vi "IO Test.vi"() -> ()   [LabVIEW 2016]
uses:
  <vilib>/rvi/Emulation/niFpgaGetClockAttributes.vi
  <vilib>/rvi/Emulation/niFpgaSctlEmulationGetInTimedLoop.vi
  <vilib>/rvi/Emulation/niFpgaEmulationReportErrorSimple.vi
  <vilib>/rvi/Emulation/niFpgaEmulationIsFPGAContextNoSignature.vi
  <vilib>/rvi/DataTransferAndStorage/Container/Common/niFpgaContainerGetUniqueNameForEmu.vi
  <vilib>/rvi/Memory/Memory_Emulation/niFpgaMemoryEmulationCacheClearOnFirstRun.vi
  <vilib>/rvi/Memory/Memory_Emulation/nirvimemoryEmulationManagerCache_MakeExclusive.vi
  <vilib>/rvi/Memory/Memory_Emulation/niFpgaMemoryEmulationValidateCache.vi
  <vilib>/rvi/Memory/Memory_Emulation/nirvimemoryEmulationManagerCache_InsertValue.vi
  <vilib>/Utility/error.llb/Clear Errors.vi
  <vilib>/rvi/Memory/Memory_Emulation/nirvimemoryEmulationManagerCache_ReleaseExclusive.vi
  <vilib>/rvi/Memory/Memory_Emulation/nirvimemoryEmulationManagerCache_GetValue.vi
  <vilib>/rvi/Memory/Memory_Emulation/nirvimemoryEmulationManagerCache_SetValue.vi
  <vilib>/rvi/Emulation/niFpgaProcessEmulError.vi
  <vilib>/rvi/eio/common/nirviEmuTemplateMethod_errors.vi
  <vilib>/rvi/Emulation/niFpgaCriticalErrorInLSC.vi
  <vilib>/rvi/DataTransferAndStorage/Container/XNode/niFpgaContainer.xnode
  <vilib>/rvi/DataTransferAndStorage/Register/Emulation/niFpgaRegisterEmulation.vi
  <vilib>/eio/EIONode/EIONode.xnode
panel:
  in  "USB Hub Relay":bool
  in  "Interlock Out":bool
  out "Interlock Sense":bool
  out "Sensor Status":u8
  in  "PAS Laser 1 Enable":bool
  in  "PAS Laser 2 Enable":bool
  in  "CRD Laser Enable":bool
  out "Temperatures":T1
  in  "Fan Voltage":i16
  in  "CRD Heater Enable":bool
  in  "PAS Heater 2":bool
  in  "PAS Heater 1":bool
  in  "Vacuum Pump":bool
  in  "Error Mode":bool
  in  "PAS Speaker Enable 2":bool
  in  "PAS Speaker Enable 1":bool
  in  "O2 Add":bool
  in  "uv light enable":bool
  in  "Fan Enable":bool
  in  "O3 Add":bool
  in  "Filter Ctl":bool
  in  "Stop":bool
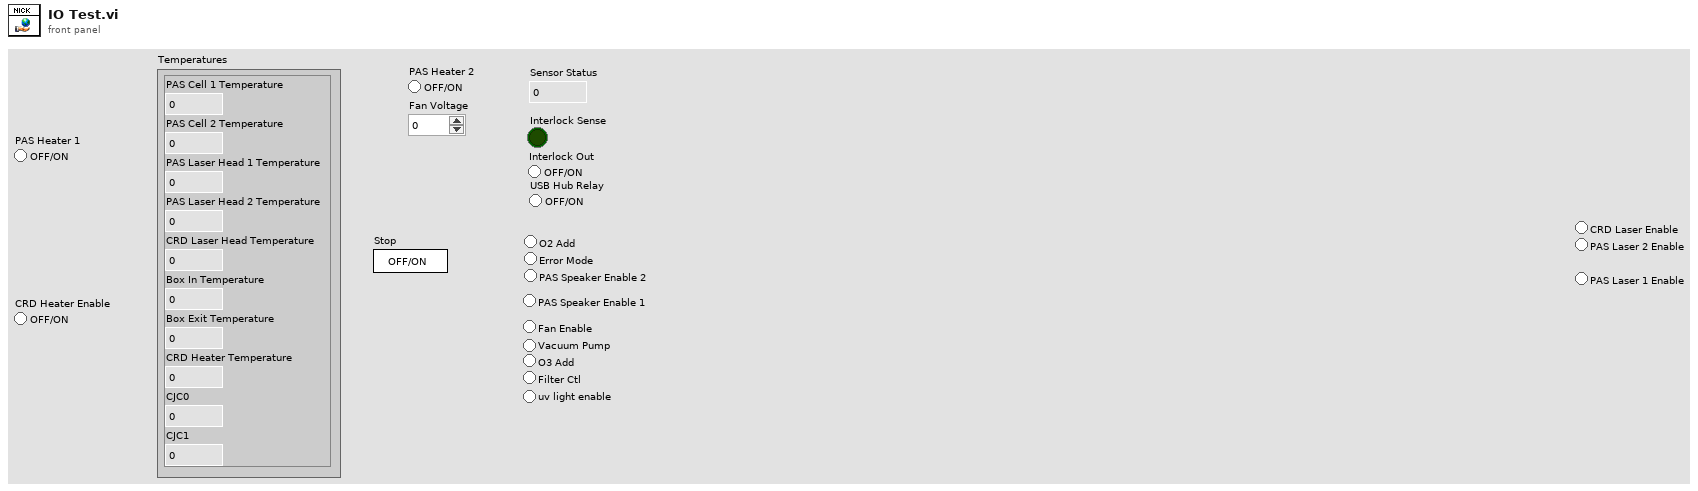
[diagram p1: front panel]
types:
  T1 = cluster{"PAS Cell 1 Temperature":fxp<+/-,24,-2>, "PAS Cell 2 Temperature":fxp<+/-,24,-2>, "PAS Laser Head 1 Temperature":fxp<+/-,24,-2>, "PAS Laser Head 2 Temperature":fxp<+/-,24,-2>, "CRD Laser Head Temperature":fxp<+/-,24,-2>, "Box In Temperature":fxp<+/-,24,-2>, "Box Exit Temperature":fxp<+/-,24,-2>, "CRD Heater Temperature":fxp<+/-,24,-2>, "CJC0":fxp<+/-,24,-2>, "CJC1":fxp<+/-,24,-2>}
  T2 = cluster{"PAS Cell 1 Temperature":fxp<+/-,24,-2>, "PAS Cell 2 Temperature":fxp<+/-,24,-2>, "PAS Laser Head 1 Temperature":fxp<+/-,24,-2>, "PAS Laser Head 2 Temperature":fxp<+/-,24,-2>, "CRD Laser Head Temperature":fxp<+/-,24,-2>, "Box In Temperature":fxp<+/-,24,-2>, "Box Exit Temperature":fxp<+/-,24,-2>, "CRD Heater Temperature":fxp<+/-,24,-2>, "Mod5/CJC0":fxp<+/-,24,-2>, "Mod5/CJC1":fxp<+/-,24,-2>}
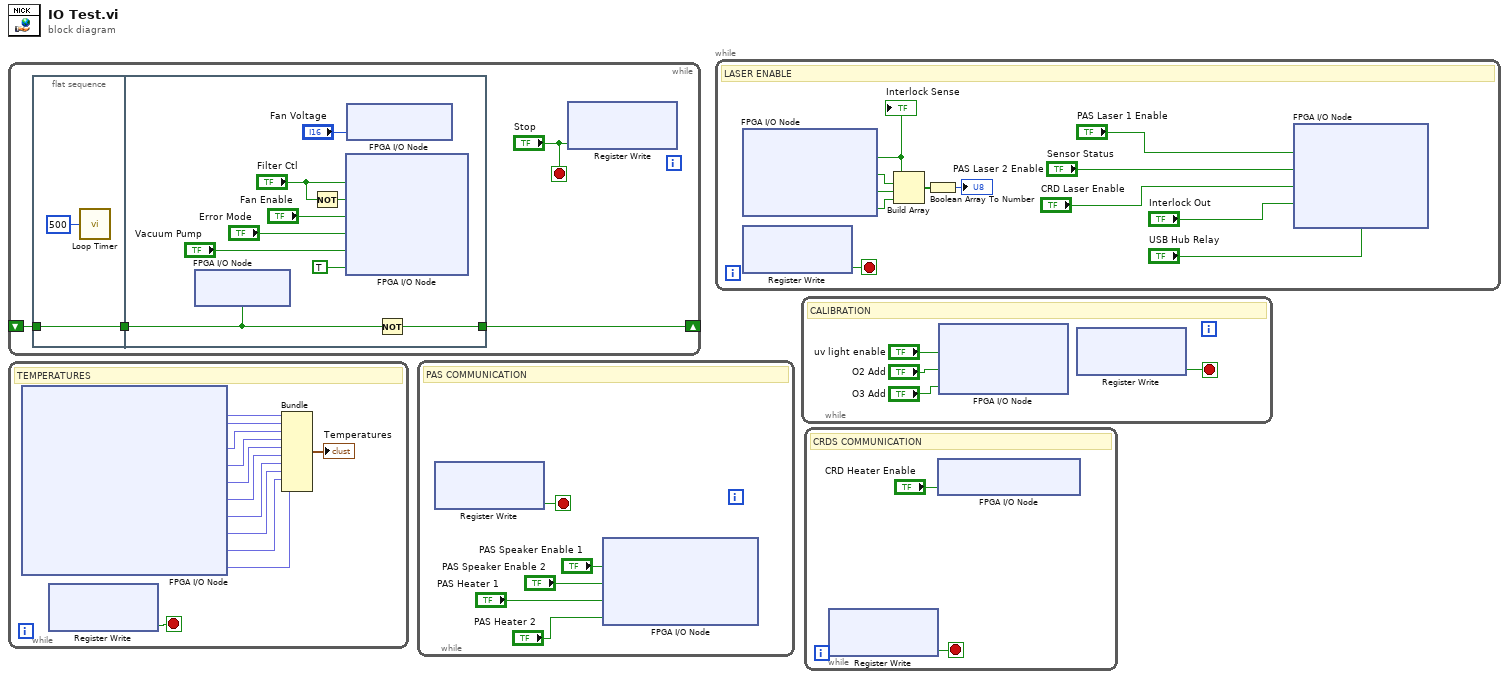
[diagram p0: block diagram]
diagram:
  n1 = while {
    shift-right: [w4] -> _
    shift-left: _ -> [w3]
    stop <- "Stop" stop-if-true
    n2 = flat-sequence {
      tunnel: w3 -> [w6]
      tunnel: [w6] -> w1
      tunnel: [w15] -> w4
      tunnel: w1 -> [w14]
      frame #0 {
        n3 = call "Loop Timer"("Count(mSec)"=u32 500) -> ()  [unwired: 1 out]
      }
      frame #1 {
        n4 = xnode "FPGA I/O Node"("Heartbeat"=w14) -> ()  [unwired: 1 in, 1 out]
        n5 = Not(x="Filter Ctl") -> (.not. x?=w12:bool)
        n6 = xnode "FPGA I/O Node"("hb 1 ctl 1"="Filter Ctl", "hb 1 ctl 2"=w12, "Fan Enable"="Fan Enable", "Error Mode"="Error Mode", "Vacuum Pump"="Vacuum Pump", "USB Hub Relay"=TRUE) -> ()  [unwired: 6 in, 6 out]
        n7 = xnode "FPGA I/O Node"("Fan Voltage"="Fan Voltage") -> ()  [unwired: 1 in, 1 out]
        n8 = Not(x=w14) -> (.not. x?=w15:bool)
      }
    }
    n9 = xnode ("Register Write")("Data"="Stop") -> ()  [unwired: 1 in, 1 out]
  }
  n10 = while {
    stop <- w27 stop-if-true
    # "TEMPERATURES"
    n11 = xnode "FPGA I/O Node"() -> ("PAS Cell 1 Temperature"=w26:fxp<+/-,24,-2>, "PAS Cell 2 Temperature"=w25:fxp<+/-,24,-2>, "PAS Laser Head 1 Temperature"=w24:fxp<+/-,24,-2>, "PAS Laser Head 2 Temperature"=w23:fxp<+/-,24,-2>, "CRD Laser Head Temperature"=w22:fxp<+/-,24,-2>, "Box In Temperature"=w21:fxp<+/-,24,-2>, "Box Exit Temperature"=w20:fxp<+/-,24,-2>, "CRD Heater Temperature"=w19:fxp<+/-,24,-2>, "Mod5/CJC0"=w18:fxp<+/-,24,-2>, "Mod5/CJC1"=w17:fxp<+/-,24,-2>)  [unwired: 10 in, 10 out]
    n12 = xnode ("Register Write")() -> ("Data"=w27:bool)  [unwired: 1 in, 1 out]
    n13 = Bundle("PAS Cell 1 Temperature"=w26, "PAS Cell 2 Temperature"=w25, "PAS Laser Head 1 Temperature"=w24, "PAS Laser Head 2 Temperature"=w23, "CRD Laser Head Temperature"=w22, "Box In Temperature"=w21, "Box Exit Temperature"=w20, "CRD Heater Temperature"=w19, "Mod5/CJC0"=w18, "Mod5/CJC1"=w17) -> (→"Temperatures":T2)  [unwired: 1 in]
  }
  n14 = while {
    stop <- w32 stop-if-true
    # "PAS COMMUNICATION"
    n15 = xnode ("Register Write")() -> ("Data"=w32:bool)  [unwired: 1 in, 1 out]
    n16 = xnode "FPGA I/O Node"("PAS Speaker Enable 1"="PAS Speaker Enable 1", "PAS Speaker Enable 2"="PAS Speaker Enable 2", "PAS Heater 1"="PAS Heater 1", "PAS Heater 2"="PAS Heater 2") -> ()  [unwired: 4 in, 4 out]
  }
  n17 = while {
    stop <- w44 stop-if-true
    # "LASER ENABLE"
    n18 = xnode "FPGA I/O Node"() -> ("Interlock Sense"=w35:bool, "hb 1 status 1"=w39:bool, "hb 1 status 2"=w38:bool, "Soft Power Down"=w37:bool)  [unwired: 4 in, 4 out]
    "Interlock Sense" <- w35
    n19 = xnode ("Register Write")() -> ("Data"=w44:bool)  [unwired: 1 in, 1 out]
    n20 = Build Array(w35, w39, w38, w37) -> (w36:bool[])
    n21 = Boolean Array To Number(Boolean array=w36) -> (number=→"Sensor Status":u8)
    n22 = xnode "FPGA I/O Node"("PAS Laser Relay 1"="PAS Laser 1 Enable", "PAS Laser Relay 2"="PAS Laser 2 Enable", "CRD Laser Enable"="CRD Laser Enable", "Interlock Sense"="Interlock Out", "USB Hub Relay"="USB Hub Relay") -> ()  [unwired: 5 in, 5 out]
  }
  n23 = while {
    stop <- w48 stop-if-true
    # "CALIBRATION"
    n24 = xnode "FPGA I/O Node"("uv light enable"="uv light enable", "Solenoid Relay 1"="O2 Add", "Solenoid Relay 2"="O3 Add") -> ()  [unwired: 3 in, 3 out]
    n25 = xnode ("Register Write")() -> ("Data"=w48:bool)  [unwired: 1 in, 1 out]
  }
  n26 = while {
    stop <- w50 stop-if-true
    # "CRDS COMMUNICATION"
    n27 = xnode ("Register Write")() -> ("Data"=w50:bool)  [unwired: 1 in, 1 out]
    n28 = xnode "FPGA I/O Node"("CRD Heater Enable"="CRD Heater Enable") -> ()  [unwired: 1 in, 1 out]
  }
